vi "System-Plot-UniversalCP.vi"(8 "Name":string, 9 "Type":T1, 10 "Dimensions":u8, 11 "ID":cluster{"ID":u32, "Element":i32[]}) -> ()   [LabVIEW 2016, in "DSI-RT.lvlib"]
uses:
  DSI-RT.lvlib
  <vilib>/addons/Software Calibration Management/xSCM/Controls/CalPoint - Type.ctl
  <vilib>/addons/Software Calibration Management/xSCM/Controls/TBL1D.ctl
  <vilib>/addons/Software Calibration Management/xSCM/Controls/TBL2D.ctl
  <vilib>/addons/Software Calibration Management/xSCM/Get/Get BOL 1D.vi
  <vilib>/addons/Software Calibration Management/xSCM/Set/Set BOL 1D.vi
  <vilib>/addons/Software Calibration Management/xSCM/Get/Get SGL 1D.vi
  <vilib>/addons/Software Calibration Management/xSCM/Set/Set SGL 1D.vi
  <vilib>/addons/Software Calibration Management/xSCM/Get/Get TLU 1D.vi
  <vilib>/addons/Software Calibration Management/xSCM/Get/Get TBL 1D.vi
  <vilib>/addons/Software Calibration Management/xSCM/Set/Set TBL 1D.vi
  <vilib>/addons/Software Calibration Management/xSCM/Get/Get BOL 2D.vi
  <vilib>/addons/Software Calibration Management/xSCM/Set/Set BOL 2D.vi
  <vilib>/addons/Software Calibration Management/xSCM/Get/Get SGL 2D.vi
  <vilib>/addons/Software Calibration Management/xSCM/Set/Set SGL 2D.vi
  <vilib>/addons/Software Calibration Management/xSCM/Get/Get TLU 2D.vi
  <vilib>/addons/Software Calibration Management/xSCM/Get/Get TBL 2D.vi
  <vilib>/addons/Software Calibration Management/xSCM/Set/Set TBL 2D.vi
  <vilib>/addons/Software Calibration Management/xSCM/SubVIs/Variant Type Index.vi
  <vilib>/addons/Software Calibration Management/xSCM/SubVIs/Variant Element By Index.vi
  <vilib>/addons/Software Calibration Management/xSCM/SubVIs/Variant Element Set.vi
  <vilib>/addons/Software Calibration Management/xSCM/Get/Get Variant.vi
  <vilib>/addons/Software Calibration Management/xSCM/SubVIs/Variant Data Index.vi
  <vilib>/addons/Software Calibration Management/xSCM/Set/Set Variant.vi
  <vilib>/addons/Software Calibration Management/xSCM/CalPoint.xnode
  <vilib>/addons/Software Calibration Management/xSCM/SCM-API.lvlib
  <vilib>/addons/Software Calibration Management/xSCM/ni_scm.dll
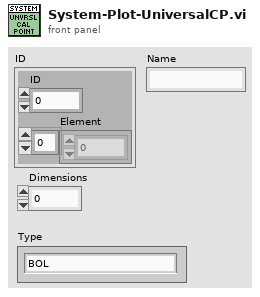
[diagram p1: front panel]
types:
  T1 = typedef "SCM-API.lvlib/CalPoint - Type.ctl" = enum8{"BOL", "U8", "U16", "U32", "U64", "I8", "I16", "I32", "I64", "SGL", "DBL", "EXT", "CSG", "CDB", "CXT", "STR", "TBL", "TLU", "CTM"}
  T2 = typedef "SCM-API.lvlib/TBL1D.ctl" = cluster{"X":sgl[], "Y":sgl[]}
  T3 = typedef "SCM-API.lvlib/TBL2D.ctl" = cluster{"X":sgl[], "Y":sgl[], "Z":sgl[][]}
  T4 = typedef "SCM-API.lvlib/TLU1D.ctl" = cluster{"X":sgl, "Y":sgl}
  T5 = typedef "SCM-API.lvlib/TLU2D.ctl" = cluster{"X":sgl, "Y":sgl, "Z":sgl}
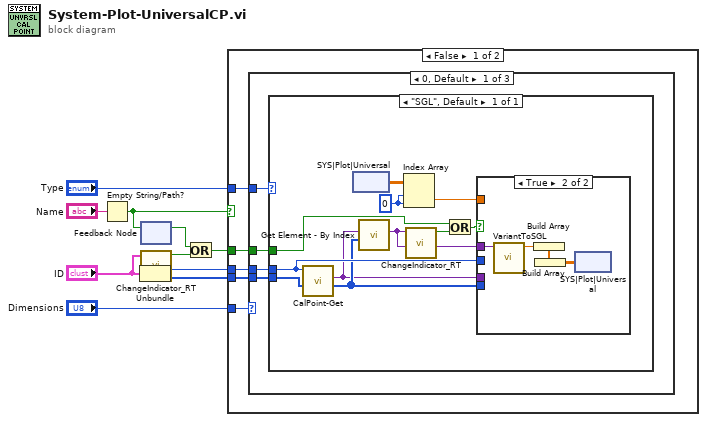
[diagram p0: block diagram]
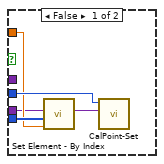
[diagram p2: hidden frame]
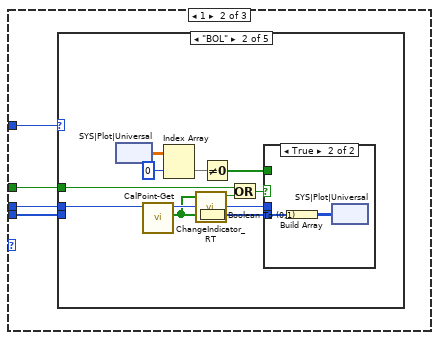
[diagram p3: hidden frame]
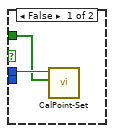
[diagram p5: hidden frame]
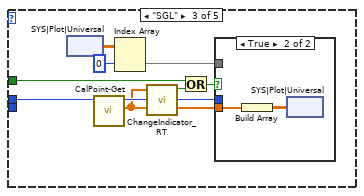
[diagram p6: hidden frame]
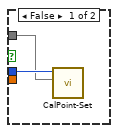
[diagram p7: hidden frame]
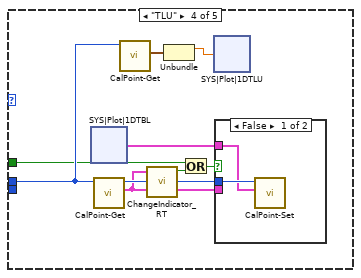
[diagram p8: hidden frame]
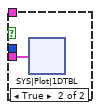
[diagram p9: hidden frame]
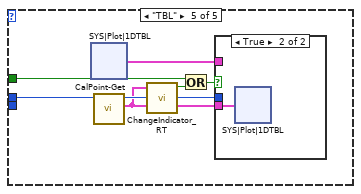
[diagram p10: hidden frame]
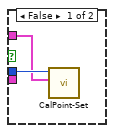
[diagram p11: hidden frame]
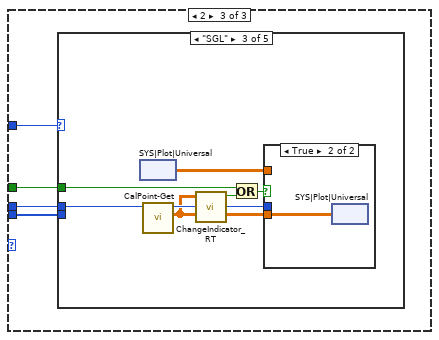
[diagram p12: hidden frame]
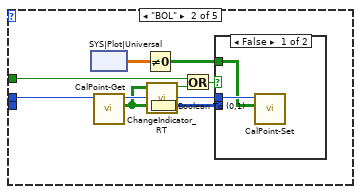
[diagram p14: hidden frame]
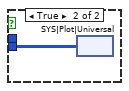
[diagram p15: hidden frame]
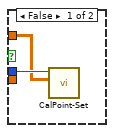
[diagram p16: hidden frame]
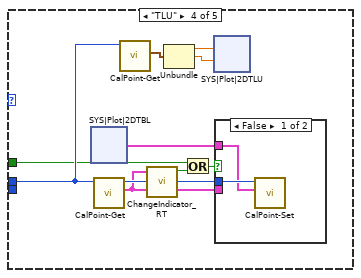
[diagram p17: hidden frame]
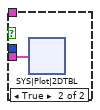
[diagram p18: hidden frame]
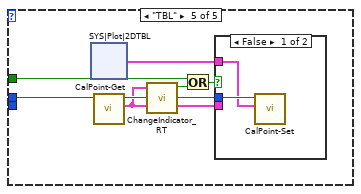
[diagram p19: hidden frame]
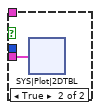
[diagram p20: hidden frame]
diagram:
  n1 = Empty String/Path?(string/path="Name") -> (empty?=w1:bool)
  n2 = Unbundle("ID") -> ("ID"=w6:u32, "Element"=w7:i32[])
  n3 = feedback-in #1(w1) -> ()
  n4 = feedback #1() -> (w2:bool)  [unwired: 1 in]
  n5 = call "ChangeIndicator_RT.vi"("Input"="ID") -> ("Change"=w4:bool)  [unwired: 9 in]
  n6 = Or(x=w2, y=w4) -> (x .or. y?=w3:bool)
  n7 = case shown="False" w1 {
    tunnel: "Type" -> [w15 _]
    tunnel: "Dimensions" -> [w14 _]
    tunnel: w6 -> [w13 _]
    tunnel: w7 -> [w12 _]
    tunnel: w3 -> [w11 _]
    frame False {
      n8 = case shown="0, Default" w14 {
        tunnel: w15 -> [w19 w59 w193]
        tunnel: w13 -> [w18 w58 w192]
        tunnel: w12 -> [w17 w57 w191]
        tunnel: w11 -> [w16 w56 w190]
        frame 0, Default {
          n9 = case shown="\"SGL\", Default" w19 {
            tunnel: w18 -> [w29]
            tunnel: w17 -> [w25]
            tunnel: w16 -> [w21]
            frame "SGL", Default {
              w27 = 0 ("index (row)")
              n10 = call-poly <vilib>:"CalPoint-Get.vi"("ID"=w29) -> ("Data"=w23:variant)  [unwired: 10 in]
              n11 = xnode "SYS|Plot|Universal"() -> ("Value"=w28:sgl[][])
              n12 = call <vilib>:"Get Element - By Index.vi"("Elements"=w25, "Variant"=w23) -> ("Element"=w24:variant)  [unwired: 8 in, 1 out]
              n13 = Index Array(array=w28, index (row)=w27, index (col)=w27) -> (element=w26:sgl)
              n14 = call "ChangeIndicator_RT.vi"("Input"=w24) -> ("Change"=w20:bool)  [unwired: 9 in]
              n15 = Or(x=w21, y=w20) -> (x .or. y?=w22:bool)
              n16 = case shown="True" w22 {
                tunnel: w29 -> [w33 _]
                tunnel: w26 -> [w31 _]
                tunnel: w24 -> [_ w38]
                tunnel: w25 -> [w32 _]
                tunnel: w23 -> [w30 _]
                frame False {
                  n17 = call <vilib>:"Set Element - By Index.vi"("Element"=w31, "Elements"=w32, "Variant"=w30) -> ("Variant"=w34:variant)  [unwired: 8 in]
                  n18 = call-poly <vilib>:"CalPoint-Set.vi"("Data"=w34, "ID"=w33) -> ()  [unwired: 10 in]
                }
                frame True {
                  n19 = call "VariantToSGL.vi"("Element"=w38) -> ("Numeric"=w35:sgl)  [unwired: 10 in]
                  n20 = Build Array(w35) -> (w37:sgl[])
                  n21 = Build Array(w37) -> (w36:sgl[][])
                  n22 = xnode "SYS|Plot|Universal"("Value"=w36) -> ()
                }
              }
            }
          }
        }
        frame 1 {
          n23 = case shown="\"BOL\"" w59 {
            tunnel: w58 -> [_ w69 w98 w127 w169]
            tunnel: w57 -> [_ _ _ _ _]
            tunnel: w56 -> [_ w62 w91 w121 w165]
            frame Default {
            }
            frame "BOL" {
              n24 = xnode "SYS|Plot|Universal"() -> ("Value"=w67:sgl[][])
              n25 = call-poly <vilib>:"CalPoint-Get.vi"("ID"=w69) -> ("Data"=w68:bool[])  [unwired: 10 in]
              n26 = Index Array(array=w67, index (row)=0) -> (element=w64:sgl[])  [unwired: 1 in]
              n27 = call "ChangeIndicator_RT.vi"("Input"=w68) -> ("Change"=w61:bool)  [unwired: 9 in]
              n28 = Boolean To (0,1)(Boolean=w68) -> (0, 1=w65:i16[])
              n29 = Not Equal To 0?(x=w64) -> (x != 0?=w66:bool[])
              n30 = Or(x=w62, y=w61) -> (x .or. y?=w60:bool)
              n31 = case shown="True" w60 {
                tunnel: w65 -> [_ w86]
                tunnel: w69 -> [w84 _]
                tunnel: w66 -> [w83 _]
                frame False {
                  n32 = call-poly <vilib>:"CalPoint-Set.vi"("Data"=w83, "ID"=w84) -> ()  [unwired: 10 in]
                }
                frame True {
                  n33 = Build Array(w86) -> (w85:i16[][])
                  n34 = xnode "SYS|Plot|Universal"("Value"=w85) -> ()
                }
              }
            }
            frame "SGL" {
              n35 = xnode "SYS|Plot|Universal"() -> ("Value"=w95:sgl[][])
              n36 = call-poly <vilib>:"CalPoint-Get.vi"("ID"=w98) -> ("Data"=w96:sgl[])  [unwired: 10 in]
              n37 = Index Array(array=w95, index (row)=0) -> (element=w93:sgl[])  [unwired: 1 in]
              n38 = call "ChangeIndicator_RT.vi"("Input"=w96) -> ("Change"=w97:bool)  [unwired: 9 in]
              n39 = Or(x=w91, y=w97) -> (x .or. y?=w92:bool)
              n40 = case shown="True" w92 {
                tunnel: w96 -> [_ w115]
                tunnel: w98 -> [w113 _]
                tunnel: w93 -> [w112 _]
                frame False {
                  n41 = call-poly <vilib>:"CalPoint-Set.vi"("Data"=w112, "ID"=w113) -> ()  [unwired: 10 in]
                }
                frame True {
                  n42 = Build Array(w115) -> (w114:sgl[][])
                  n43 = xnode "SYS|Plot|Universal"("Value"=w114) -> ()
                }
              }
            }
            frame "TLU" {
              n44 = xnode "SYS|Plot|1DTBL"() -> ("Value"=w125:T2)
              n45 = call-poly <vilib>:"CalPoint-Get.vi"("ID"=w127) -> ("Data"=w126:T2)  [unwired: 10 in]
              n46 = call-poly <vilib>:"CalPoint-Get.vi"("ID"=w127) -> ("Data"=w124:T4)  [unwired: 10 in]
              n47 = call "ChangeIndicator_RT.vi"("Input"=w126) -> ("Change"=w122:bool)  [unwired: 9 in]
              n48 = Unbundle(w124) -> ("X"=w123:sgl)  [unwired: 1 out]
              n49 = Or(x=w121, y=w122) -> (x .or. y?=w120:bool)
              n50 = xnode "SYS|Plot|1DTLU"("X Index"=w123) -> ()  [unwired: 1 out]
              n51 = case shown="False" w120 {
                tunnel: w126 -> [_ w159]
                tunnel: w127 -> [w158 _]
                tunnel: w125 -> [w157 _]
                frame False {
                  n52 = call-poly <vilib>:"CalPoint-Set.vi"("Data"=w157, "ID"=w158) -> ()  [unwired: 10 in]
                }
                frame True {
                  n53 = xnode "SYS|Plot|1DTBL"("Value"=w159) -> ()
                }
              }
            }
            frame "TBL" {
              n54 = xnode "SYS|Plot|1DTBL"() -> ("Value"=w167:T2)
              n55 = call-poly <vilib>:"CalPoint-Get.vi"("ID"=w169) -> ("Data"=w168:T2)  [unwired: 10 in]
              n56 = call "ChangeIndicator_RT.vi"("Input"=w168) -> ("Change"=w166:bool)  [unwired: 9 in]
              n57 = Or(x=w165, y=w166) -> (x .or. y?=w164:bool)
              n58 = case shown="True" w164 {
                tunnel: w168 -> [_ w185]
                tunnel: w169 -> [w184 _]
                tunnel: w167 -> [w183 _]
                frame False {
                  n59 = call-poly <vilib>:"CalPoint-Set.vi"("Data"=w183, "ID"=w184) -> ()  [unwired: 10 in]
                }
                frame True {
                  n60 = xnode "SYS|Plot|1DTBL"("Value"=w185) -> ()
                }
              }
            }
          }
        }
        frame 2 {
          n61 = case shown="\"SGL\"" w193 {
            tunnel: w192 -> [_ w201 w227 w256 w312]
            tunnel: w191 -> [_ _ _ _ _]
            tunnel: w190 -> [_ w195 w223 w249 w308]
            frame Default {
            }
            frame "BOL" {
              n62 = xnode "SYS|Plot|Universal"() -> ("Value"=w199:sgl[][])
              n63 = call-poly <vilib>:"CalPoint-Get.vi"("ID"=w201) -> ("Data"=w200:bool[][])  [unwired: 10 in]
              n64 = Not Equal To 0?(x=w199) -> (x != 0?=w198:bool[][])
              n65 = call "ChangeIndicator_RT.vi"("Input"=w200) -> ("Change"=w196:bool)  [unwired: 9 in]
              n66 = Boolean To (0,1)(Boolean=w200) -> (0, 1=w197:i16[][])
              n67 = Or(x=w195, y=w196) -> (x .or. y?=w194:bool)
              n68 = case shown="False" w194 {
                tunnel: w197 -> [_ w217]
                tunnel: w201 -> [w216 _]
                tunnel: w198 -> [w215 _]
                frame False {
                  n69 = call-poly <vilib>:"CalPoint-Set.vi"("Data"=w215, "ID"=w216) -> ()  [unwired: 10 in]
                }
                frame True {
                  n70 = xnode "SYS|Plot|Universal"("Value"=w217) -> ()
                }
              }
            }
            frame "SGL" {
              n71 = xnode "SYS|Plot|Universal"() -> ("Value"=w225:sgl[][])
              n72 = call-poly <vilib>:"CalPoint-Get.vi"("ID"=w227) -> ("Data"=w226:sgl[][])  [unwired: 10 in]
              n73 = call "ChangeIndicator_RT.vi"("Input"=w226) -> ("Change"=w224:bool)  [unwired: 9 in]
              n74 = Or(x=w223, y=w224) -> (x .or. y?=w222:bool)
              n75 = case shown="True" w222 {
                tunnel: w226 -> [_ w243]
                tunnel: w227 -> [w242 _]
                tunnel: w225 -> [w241 _]
                frame False {
                  n76 = call-poly <vilib>:"CalPoint-Set.vi"("Data"=w241, "ID"=w242) -> ()  [unwired: 10 in]
                }
                frame True {
                  n77 = xnode "SYS|Plot|Universal"("Value"=w243) -> ()
                }
              }
            }
            frame "TLU" {
              n78 = xnode "SYS|Plot|2DTBL"() -> ("Value"=w254:T3)
              n79 = call-poly <vilib>:"CalPoint-Get.vi"("ID"=w256) -> ("Data"=w255:T3)  [unwired: 10 in]
              n80 = call-poly <vilib>:"CalPoint-Get.vi"("ID"=w256) -> ("Data"=w253:T5)  [unwired: 10 in]
              n81 = call "ChangeIndicator_RT.vi"("Input"=w255) -> ("Change"=w250:bool)  [unwired: 9 in]
              n82 = Unbundle(w253) -> ("X"=w252:sgl, "Y"=w251:sgl)  [unwired: 1 out]
              n83 = Or(x=w249, y=w250) -> (x .or. y?=w248:bool)
              n84 = xnode "SYS|Plot|2DTLU"("Y Index"=w251, "X Index"=w252) -> ()  [unwired: 1 out]
              n85 = case shown="False" w248 {
                tunnel: w255 -> [_ w302]
                tunnel: w256 -> [w301 _]
                tunnel: w254 -> [w300 _]
                frame False {
                  n86 = call-poly <vilib>:"CalPoint-Set.vi"("Data"=w300, "ID"=w301) -> ()  [unwired: 10 in]
                }
                frame True {
                  n87 = xnode "SYS|Plot|2DTBL"("Value"=w302) -> ()
                }
              }
            }
            frame "TBL" {
              n88 = xnode "SYS|Plot|2DTBL"() -> ("Value"=w310:T3)
              n89 = call-poly <vilib>:"CalPoint-Get.vi"("ID"=w312) -> ("Data"=w311:T3)  [unwired: 10 in]
              n90 = call "ChangeIndicator_RT.vi"("Input"=w311) -> ("Change"=w309:bool)  [unwired: 9 in]
              n91 = Or(x=w308, y=w309) -> (x .or. y?=w307:bool)
              n92 = case shown="False" w307 {
                tunnel: w311 -> [_ w328]
                tunnel: w312 -> [w327 _]
                tunnel: w310 -> [w326 _]
                frame False {
                  n93 = call-poly <vilib>:"CalPoint-Set.vi"("Data"=w326, "ID"=w327) -> ()  [unwired: 10 in]
                }
                frame True {
                  n94 = xnode "SYS|Plot|2DTBL"("Value"=w328) -> ()
                }
              }
            }
          }
        }
      }
    }
    frame True {
      n95 = xnode "SYS|Plot|Universal"("Value"=sgl[][] []) -> ()
    }
  }
